vi "cryo_comm.vi"(8 "error in (no error)":errorcluster, 10 "String":string, 11 "TCP Network Connection in":refnum<k5>) -> (0 "error out 2":errorcluster, 1 "Message [2] (return value)":string, 2 "Message [1]":string, 3 "Message [0]":string)   [LabVIEW 2023]
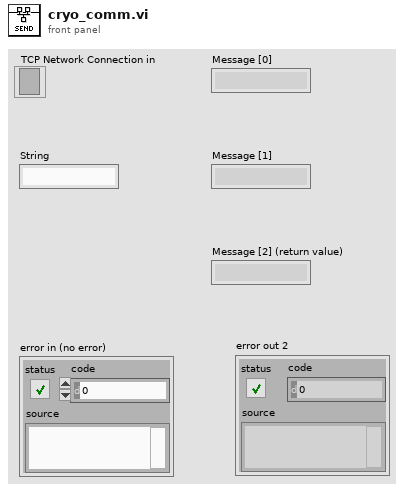
[diagram p1: front panel]
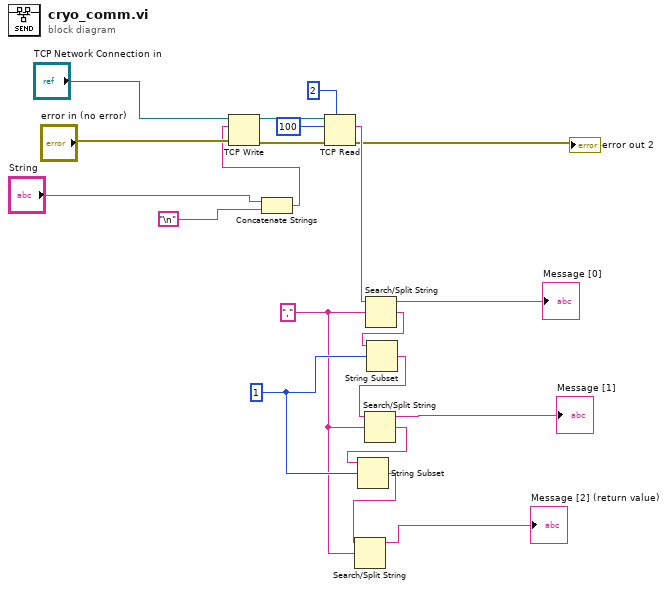
[diagram p0: block diagram]
diagram:
  w20 = 1
  w12 = ","
  n1 = Concatenate Strings("String", "\n") -> (w6:string)
  n2 = TCP Write(connection ID="TCP Network Connection in", data in=w6, error in (no error)="error in (no error)") -> (connection ID out=w7:refnum<k5>, error out=w8:errorcluster)  [unwired: 1 in, 1 out]
  n3 = TCP Read(connection ID=w7, bytes to read=100, error in (no error)=w8, 7:2) -> (data out=w11:string, error out=→"error out 2":errorcluster)  [unwired: 1 in, 1 out]
  n4 = Search/Split String(string=w11, search string/char (-)=w12) -> (substring before match=→"Message [0]":string, match + rest of string=w16:string)  [unwired: 1 in, 1 out]
  n5 = String Subset(string=w16, offset (0)=w20) -> (substring=w17:string)  [unwired: 1 in]
  n6 = Search/Split String(string=w17, search string/char (-)=w12) -> (substring before match=→"Message [1]":string, match + rest of string=w18:string)  [unwired: 1 in, 1 out]
  n7 = String Subset(string=w18, offset (0)=w20) -> (substring=w19:string)  [unwired: 1 in]
  n8 = Search/Split String(string=w19, search string/char (-)=w12) -> (substring before match=→"Message [2] (return value)":string)  [unwired: 1 in, 2 out]
